vi "Init_PM.vi"(8 "error in (no error)":errorcluster {"code" format="%.0x"}) -> (0 "error out":errorcluster, 1 "Sensor Name":string, 3 "instrument handle out":refnum<visa-resource-name>)   [LabVIEW 2018]
panel:
  in  "instrument handle in":refnum<visa-resource-name>
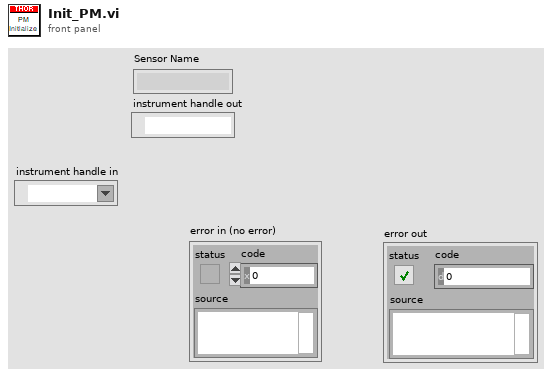
[diagram p1: front panel]
types:
  T1 = enum16{"Init", "Set-Get Avg", "Set-Get Wavelength", "Do measure"}
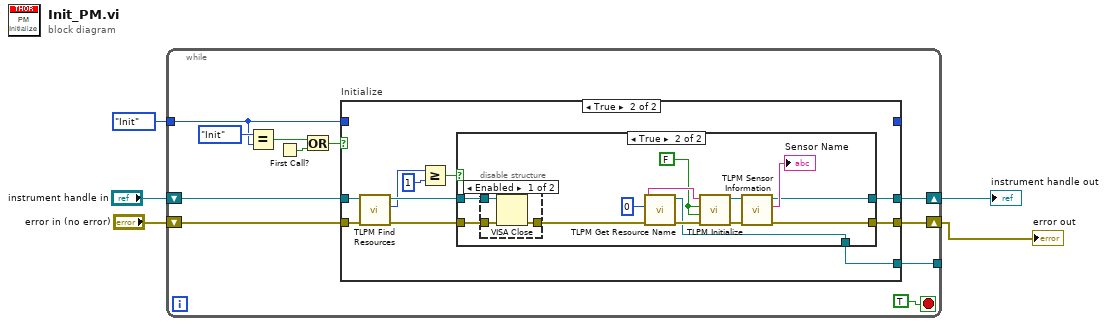
[diagram p0: block diagram]
diagram:
  n1 = while {
    shift-right: [w8] -> w2
    shift-left: "error in (no error)" -> [w14]
    tunnel: T1."Init" -> [w9]
    shift-right: [w7] -> w1
    shift-left: "instrument handle in" -> [w15]
    tunnel: [w6] -> _
    stop <- TRUE stop-if-true
    n2 = Equal?(x=T1."Init" ("y"), y=w9) -> (x = y?=w13:bool)
    n3 = First Call?() -> (First Call?: T/F=w12:bool)
    n4 = Or(x=w13, y=w12) -> (x .or. y?=w11:bool)
    n5 = case "Initialize" shown="True" w11 {
      tunnel: w15 -> [w17 w29]
      tunnel: [w18 w27] -> w8
      tunnel: w14 -> [w18 w23]
      tunnel: [w19 _] -> _
      tunnel: w9 -> [w19 _]
      tunnel: [w17 w28] -> w7
      tunnel: [_ w20] -> w6
      frame False {
      }
      frame True {
        n6 = call "TLPM Find Resources.vi"("error in (no error)"=w23, "instrument handle"=w29) -> ("error out"=w22:errorcluster, "Resource Count"=w21:u32, "instrument handle out"=w24:refnum<visa-resource-name>)  [unwired: 7 in]
        n7 = Greater Or Equal?(x=w21, y=u32 1) -> (x >= y?=w25:bool)
        n8 = case shown="True" w25 {
          tunnel: w22 -> [w30 w33]
          tunnel: w24 -> [w31 w34]
          tunnel: [w31 w37] -> w28
          tunnel: [w30 w36] -> w27
          tunnel: [_ w35] -> w20
          frame False {
          }
          frame True {
            w42 = FALSE ("ID Query (Do Query)")
            n9 = disable-structure shown="Enabled" {
              disable-tunnel: w34 -> [w47 _]
              disable-tunnel: w33 -> [w46 w48]
              disable-tunnel: [w45 w48] -> w32
              frame Enabled {
                n10 = VISA Close(VISA resource name=w47, error in (no error)=w46) -> (error out=w45:errorcluster)
              }
              frame Disabled {
              }
            }
            n11 = call "TLPM Get Resource Name.vi"("error in (no error)"=w32, "Index (0)"=u32 0) -> ("error out"=w44:errorcluster, "instrument handle out"=w35:refnum<visa-resource-name>, "Resource Name"=w43:string)  [unwired: 7 in]
            n12 = call "TLPM Initialize.vi"("error in (no error)"=w44, "Reset Device (Reset Device)"=w42, "ID Query (Do Query)"=w42, "resource name"=w43) -> ("error out"=w40:errorcluster, "instrument handle out"=w39:refnum<visa-resource-name>)  [unwired: 6 in]
            n13 = call "TLPM Sensor Information.vi"("error in (no error)"=w40, "instrument handle"=w39) -> ("error out"=w36:errorcluster, "Sensor Name"=→"Sensor Name":string, "instrument handle out"=w37:refnum<visa-resource-name>)  [unwired: 2 in, 5 out]
          }
        }
      }
    }
  }
  "error out" <- w2
  "instrument handle out" <- w1
